vi "Find Event Structure from Case Structure.vi"(8 "error in (no error)":errorcluster, 11 "CaseStructure":refnum<vi>) -> (0 "error out":errorcluster, 1 "EvntStruct Refnum":refnum<vi>)   [LabVIEW 2020, in "JKI State Machine API.lvlib" / "JKI SM.lvclass"]
uses:
  JKI SM.lvclass
  JKI SM.lvclass/JKI SM.ctl
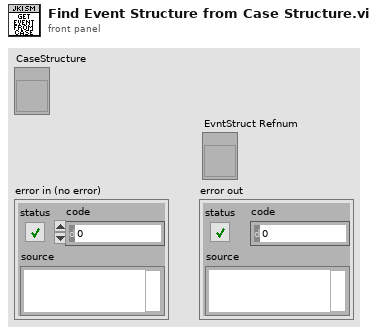
[diagram p1: front panel]
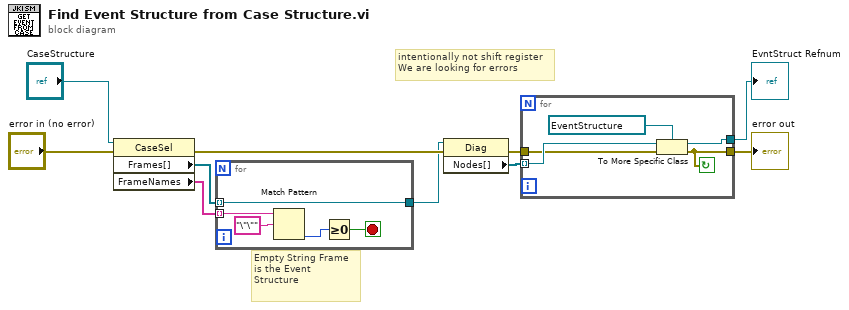
[diagram p0: block diagram]
diagram:
  # "Empty String Frame is the Event Structure"
  # "intentionally not shift register\nWe are looking for errors"
  n1 = property class="CaseSel"(reference="CaseStructure", error in="error in (no error)") -> (error out=w7:errorcluster, "Frames[]"=w2:refnum<vi>[], "FrameNames"=w3:string[])  [unwired: 1 out]
  n2 = for {
    tunnel: w3 -> [w15] mode=indexing
    tunnel: w2 -> [w11] mode=indexing
    tunnel: [w11] -> w1
    stop <- w12 stop-if-true
    n3 = Match Pattern(string=w15, regular expression="\"\"") -> (offset past match=w13:i32)  [unwired: 1 in, 3 out]
    n4 = Greater Or Equal To 0?(x=w13) -> (x >= 0?=w12:bool)
  }
  n5 = property class="Diag"(reference=w1, error in=w7) -> (error out=w5:errorcluster, "Nodes[]"=w8:refnum<vi>[])  [unwired: 1 out]
  n6 = for {
    tunnel: w8 -> [w19] mode=indexing
    tunnel: [w18] -> w6
    tunnel: w5 -> [w17]
    tunnel: [w16] -> w4
    stop <- w16 continue-if-true
    n7 = To More Specific Class(target class=refnum<vi> refnum ("EvntStruct Refnum"), reference=w19, error in=w17) -> (specific class reference=w18:refnum<vi>, error out=w16:errorcluster)
  }
  "error out" <- w4
  "EvntStruct Refnum" <- w6
